vi "SVT Audio Filter (1 Ch).vi"(6 "reset filter (F)":bool, 8 "error in (no error)":errorcluster, 10 "filter type":u16(ring) items=["Linear"=0, "AES17 20 kHz Lowpass"=17, "AES17 40 kHz Lowpass"=18, "AES17 20 kHz Highpass"=19, "AES17 40 kHz Highpass"=20], 11 "scaled signal [EU]":waveform(dbl)) -> (0 "error out":errorcluster, 1 "phase response":cluster{"f0":dbl, "df":dbl, "Phase":dbl[]}, 2 "magnitude response":cluster{"f0":dbl, "df":dbl, "Mag":dbl[]}, 3 "filtered signal [EU]":waveform(dbl))   [LabVIEW 2017, in "SoundVib_AudioFilter.lvlib"]
doc: "Applies the selected audio weighting filter to the <B>scaled signal [EU]</B>. Wire data to the <B>scaled signal [EU]</B> input to determine the polymorphic instance to use or manually select the instance."
uses:
  <vilib>/addons/Sound and Vibration/svt_Weighting/SoundVib_AudioFilter.lvlib
  <vilib>/addons/_NISVFA/_Shared subVIs/Common/svc_Check for Waveform Parameter Continuity (no state).vi
  <vilib>/addons/_NISVFA/_Shared subVIs/Common/svc_Get SV Channel Info.vi
  <vilib>/addons/_NISVFA/_Shared subVIs/Common/svc_Engineering Units to Unit Label.vi
  <vilib>/addons/_NISVFA/_Shared subVIs/Common/svc_Unit Label to Engineering Units.vi
  <vilib>/Analysis/NI_AALBase.lvlib
  <vilib>/measure/NI_MAPro.lvlib
  <vilib>/measure/NI_MABase.lvlib
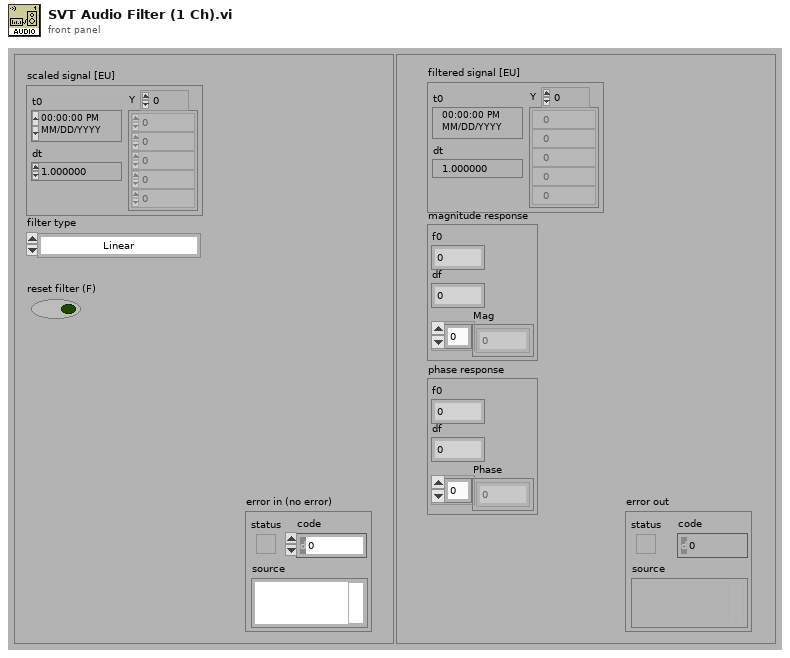
[diagram p1: front panel]
types:
  T1 = cluster{"dt":bool, "t0 continuity":bool, "array length":bool, "channel info":bool, "name":bool}
  T2 = enum32{"Lowpass", "Highpass", "Bandpass", "Bandstop"}
  T3 = typedef "svc_Weighting Filter Text Ring.ctl" = u16
  T4 = cluster{"filter structure":enum32{"IIR 2nd Order", "IIR 4th Order"}, "Reverse Coefficients":dbl[], "Forward Coefficients":dbl[]}
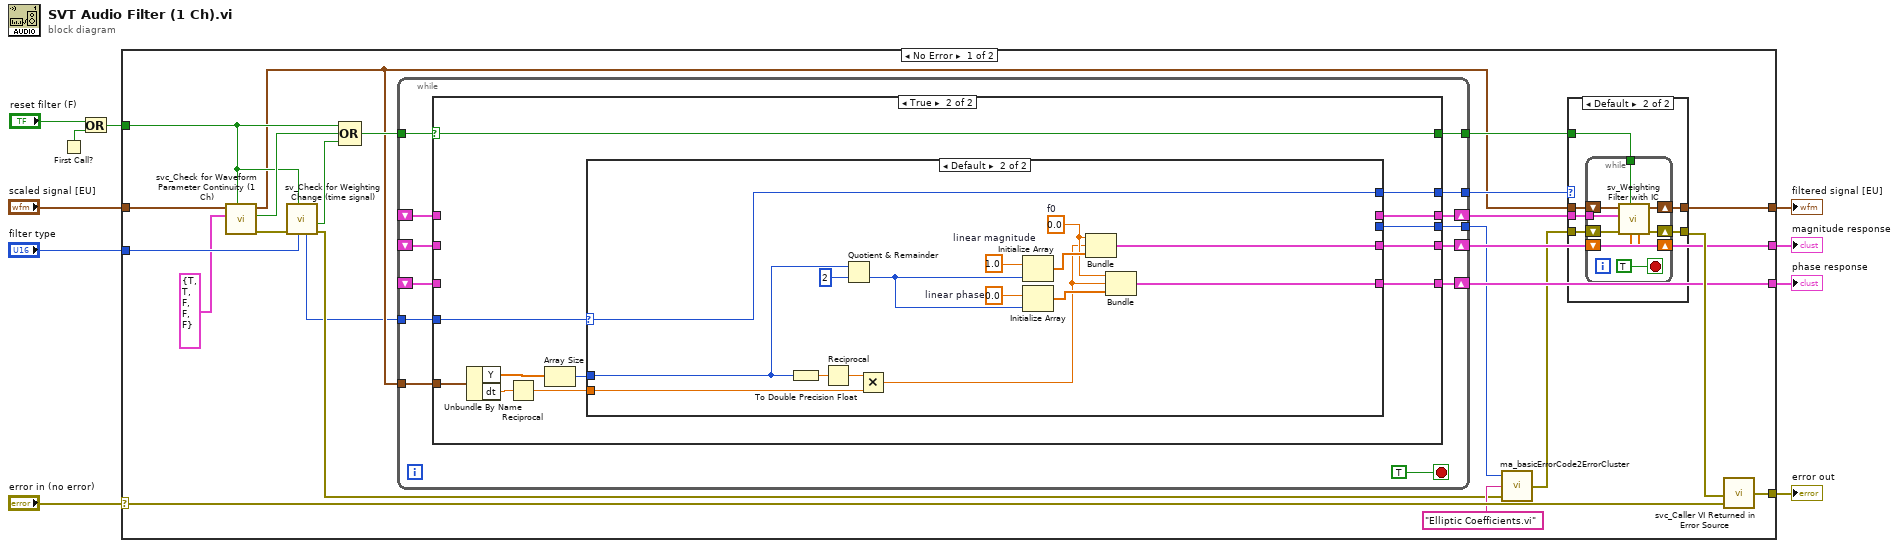
[diagram p0: block diagram]
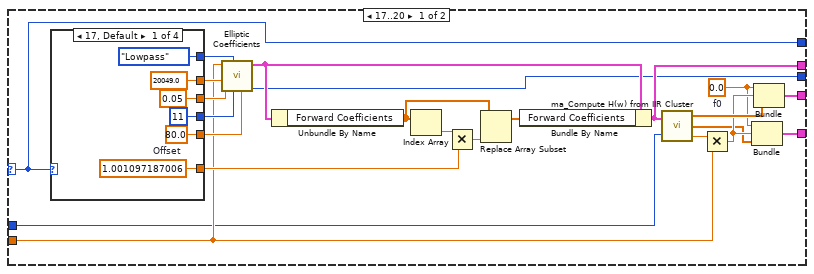
[diagram p4: hidden frame]
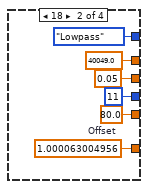
[diagram p5: hidden frame]
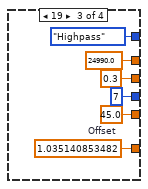
[diagram p6: hidden frame]
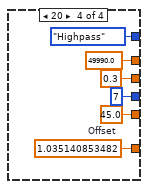
[diagram p7: hidden frame]
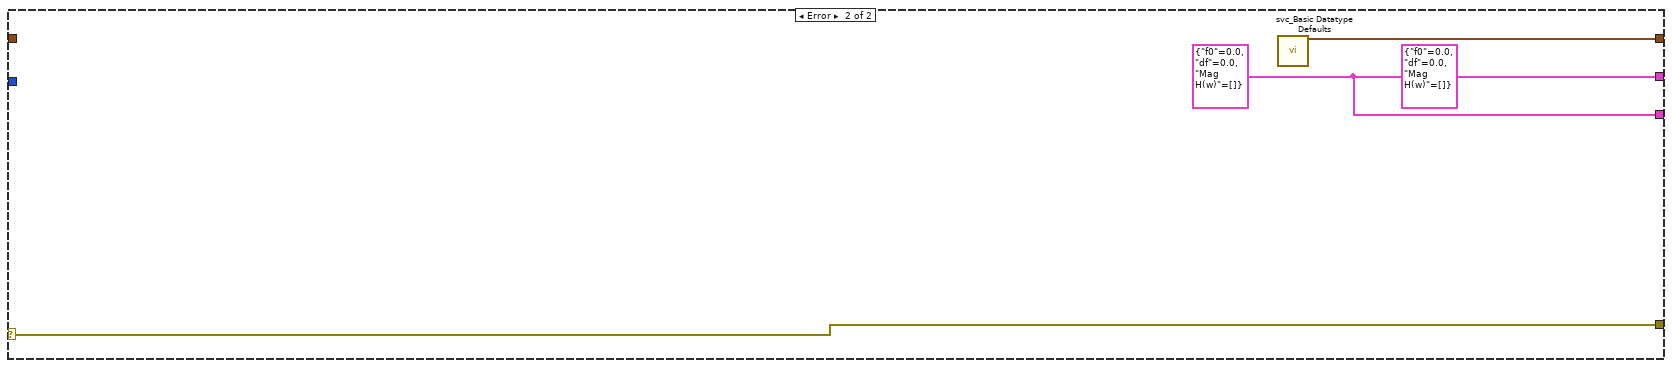
[diagram p8: hidden frame]
diagram:
  n1 = First Call?() -> (First Call?: T/F=w3:bool)
  n2 = Or(x="reset filter (F)", y=w3) -> (x .or. y?=w7:bool)
  n3 = case shown="No Error" "error in (no error)" {
    selector: "error in (no error)" -> [w17 w145]
    tunnel: [w20 w145] -> w10
    tunnel: [w18 w144] -> w9
    tunnel: "scaled signal [EU]" -> [w25 _]
    tunnel: w7 -> [w24 _]
    tunnel: "filter type" -> [w21 _]
    tunnel: [w22 w143] -> w2
    tunnel: [w23 w143] -> w1
    frame No Error {
      n4 = call <vilib>:"svc_Check for Waveform Parameter Continuity (1 Ch).vi"("restart averaging (F)"=w24, "checks for channel parameter change"=T1 {"dt"=TRUE, "t0 continuity"=TRUE, "array length"=FALSE, "channel info"=FALSE, "name"=FALSE}, "scaled signal [EU]"=w25) -> ("error out"=w30:errorcluster, "waveform parameter changed"=w32:bool, "dup scaled signal [EU]"=w19:waveform(dbl))  [unwired: 3 in, 3 out]
      n5 = call <vilib>:"sv_Check for Weighting Change (time signal).vi"("weighting"=w21, "reset (in)"=w24, "error in (no error)"=w30) -> ("error out"=w15:errorcluster, "weighting has changed"=w33:bool, "dup weighting"=w12:T3)  [unwired: 6 in]
      n6 = Compound Arithmetic op=OR(w24, w32, w33) -> (w31:bool)
      n7 = while {
        shift-right: [w62] -> w29
        shift-left: _ -> [w63]
        shift-right: [w61] -> w22
        shift-left: _ -> [w58]
        shift-right: [w60] -> w23
        shift-left: _ -> [w59]
        tunnel: [w57] -> w28
        tunnel: w12 -> [w56]
        tunnel: [w55] -> w27
        tunnel: w31 -> [w54]
        tunnel: w19 -> [w53]
        tunnel: [w51] -> w14
        stop <- TRUE stop-if-true
        n8 = case shown="True" w54 {
          selector: w54 -> [w65 w76]
          tunnel: w53 -> [_ w80]
          tunnel: w63 -> [w68 _]
          tunnel: [w68 w79] -> w62
          tunnel: [w67 w78] -> w61
          tunnel: [w66 w77] -> w60
          tunnel: w59 -> [w66 _]
          tunnel: w58 -> [w67 _]
          tunnel: [w65 w76] -> w57
          tunnel: w56 -> [w64 w74]
          tunnel: [w64 w75] -> w55
          tunnel: [_ w69] -> w51
          frame False {
            # "Filter is not reset"
          }
          frame True {
            n9 = Unbundle By Name(w80) -> ("Y"=w71:dbl[], "dt"=w73:dbl)
            n10 = Reciprocal(x=w73) -> (1/x=w72:dbl)
            n11 = Array Size(array=w71) -> (size(s)=w70:i32)
            n12 = case shown="Default" w74 {
              selector: w74 -> [w90 w136]
              tunnel: w72 -> [w83 w134]
              tunnel: [w97 _] -> w79
              tunnel: [w95 w137] -> w78
              tunnel: [w91 w138] -> w77
              tunnel: [w90 w136] -> w75
              tunnel: w70 -> [w82 w128]
              tunnel: [w81 _] -> w69
              frame 17..20 {
                w92 = 0.0  # f0
                n13 = case shown="17, Default" w90 {
                  tunnel: [w109 w115 w121 w127] -> w102
                  tunnel: [T2."Lowpass" ("filter type") T2."Lowpass" ("filter type") T2."Highpass" ("filter type") T2."Highpass" ("filter type")] -> w89
                  tunnel: [20049.0 ("low cutoff freq: fl") 40049.0 ("low cutoff freq: fl") 24990.0 ("low cutoff freq: fl") 49990.0 ("low cutoff freq: fl")] -> w85
                  tunnel: [11 ("order") 11 ("order") 7 ("order") 7 ("order")] -> w87
                  tunnel: [80.0 ("stopband attenuation (dB)") 80.0 ("stopband attenuation (dB)") 45.0 ("stopband attenuation (dB)") 45.0 ("stopband attenuation (dB)")] -> w86
                  tunnel: [0.05 ("low cutoff freq: fl") 0.05 ("low cutoff freq: fl") 0.3 ("low cutoff freq: fl") 0.3 ("low cutoff freq: fl")] -> w84
                  frame 17, Default {
                    w109 = 1.001097187006  # Offset
                  }
                  frame 18 {
                    w115 = 1.000063004956  # Offset
                  }
                  frame 19 {
                    w121 = 1.035140853482  # Offset
                  }
                  frame 20 {
                    w127 = 1.035140853482  # Offset
                  }
                }
                n14 = call <vilib>:"Elliptic Coefficients.vi"("stopband attenuation (dB)"=w86, "order"=w87, "filter type"=w89, "passband ripple (dB)"=w84, "low cutoff freq: fl"=w85, "sampling freq: fs"=w83) -> ("error"=w81:i32, "IIR Filter Cluster"=w88:T4)  [unwired: 4 in]
                n15 = Unbundle By Name(w88) -> ("Forward Coefficients"=w101:dbl[])
                n16 = Index Array(array=w101) -> (element=w103:dbl)  [unwired: 1 in]
                n17 = Multiply(x=w103, y=w102) -> (x*y=w100:dbl)
                n18 = Replace Array Subset(array=w101, new element=w100) -> (w99:dbl[])  [unwired: 1 in]
                n19 = Bundle By Name(cluster=w88, "Forward Coefficients"=w99) -> (w97:T4)
                n20 = call <vilib>:"ma_Compute H(w) from IIR Cluster.vi"("IIR Filter Cluster"=w97, "FFT size"=w82) -> ("Mag H(w)"=w96:dbl[], "Phase H(w)"=w93:dbl[], "df"=w98:dbl)
                n21 = Multiply(x=w98, y=w83) -> (x*y=w94:dbl)
                n22 = Bundle("f0"=w92, w94, "Phase H(w)"=w93) -> (w91:cluster{"f0":dbl, dbl, "Phase H(w)":dbl[]})  [unwired: 1 in]
                n23 = Bundle("f0"=w92, w94, "Mag H(w)"=w96) -> (w95:cluster{"f0":dbl, dbl, "Mag H(w)":dbl[]})  [unwired: 1 in]
              }
              frame Default {
                w142 = 1.0  # linear magnitude
                w140 = 0.0  # linear phase
                w133 = 0.0  # f0
                n24 = To Double Precision Float(number=w128) -> (double precision float=w131:dbl)
                n25 = Reciprocal(x=w131) -> (1/x=w135:dbl)
                n26 = Quotient & Remainder(x=w128, y=2) -> (floor(x/y)=w129:i32)  [unwired: 1 out]
                n27 = Multiply(x=w135, y=w134) -> (x*y=w132:dbl)
                n28 = Initialize Array(w142, w129) -> (w139:dbl[])
                n29 = Initialize Array(w140, w129) -> (w141:dbl[])
                n30 = Bundle("f0"=w133, w132, w139) -> (w137:cluster{"f0":dbl, dbl, dbl[]})  [unwired: 1 in]
                n31 = Bundle("f0"=w133, w132, w141) -> (w138:cluster{"f0":dbl, dbl, dbl[]})  [unwired: 1 in]
              }
            }
          }
        }
      }
      n32 = call <vilib>:"ma_basicErrorCode2ErrorCluster.vi"("error in (no error)"=w15, "subVI name"="Elliptic Coefficients.vi", "Error Code"=w14) -> ("error out"=w13:errorcluster)
      n33 = case shown="Default" w27 {
        tunnel: [w35 w41] -> w18
        tunnel: w29 -> [_ w40]
        tunnel: w28 -> [_ w39]
        tunnel: w19 -> [w35 w36]
        tunnel: w13 -> [w34 w38]
        tunnel: [w34 w37] -> w26
        frame 0 {
        }
        frame Default {
          n34 = while {
            tunnel: w40 -> [w49]
            tunnel: w39 -> [w48]
            shift-right: [w50] -> w41
            shift-left: w36 -> [w45]
            shift-right: [w46] -> w37
            shift-left: w38 -> [w47]
            shift-right: [w44] -> _
            shift-left: _ -> [w43]
            stop <- TRUE stop-if-true
            n35 = call <vilib>:"sv_Weighting Filter with IC.vi"("Initial Filter State"=w43, "error in (no error)"=w47, "reset filter (F)"=w48, "filter coefficients"=w49, "signal [V]"=w45) -> ("error out"=w46:errorcluster, "filtered signal [EU]"=w50:waveform(dbl), "Final Filter State"=w44:dbl[])  [unwired: 4 in]
          }
        }
      }
      n36 = call <vilib>:"svc_Caller VI Returned in Error Source.vi"("warning input to caller"=w17, "error in (no error)"=w26) -> ("error out"=w20:errorcluster)  [unwired: 3 in]
    }
    frame Error {
      w143 = cluster{"f0":dbl, "df":dbl, "Mag H(w)":dbl[]} {"f0"=0.0, "df"=0.0, "Mag H(w)"=[]} ("magnitude H(w)")
      (unwired) cluster{"f0":dbl, "df":dbl, "Mag H(w)":dbl[]} {"f0"=0.0, "df"=0.0, "Mag H(w)"=[]} ("magnitude H(w)")
      n37 = call <vilib>:"svc_Basic Datatype Defaults.vi"() -> ("empty waveform"=w144:waveform(dbl))  [unwired: 7 in, 12 out]
    }
  }
  "error out" <- w10
  "filtered signal [EU]" <- w9
  "magnitude response" <- w2
  "phase response" <- w1
